vi "水温校准.vi"() -> ()   [LabVIEW 2016, in "斯坦道多参数.lvlib"]
uses:
  <vilib>/Utility/config.llb/NI_LVConfig.lvlib
panel:
  in  "补偿后温度值":dbl
  out "电极温度读值":dbl
  in  "温度偏移补偿":dbl
  in  "温度电极选择":enum16{"pH电极", "电导率电极", "溶解氧电极", "浊度电极"}(ring)
  # "温度电极设定"
  # "℃"
  # "℃"
  # "℃"
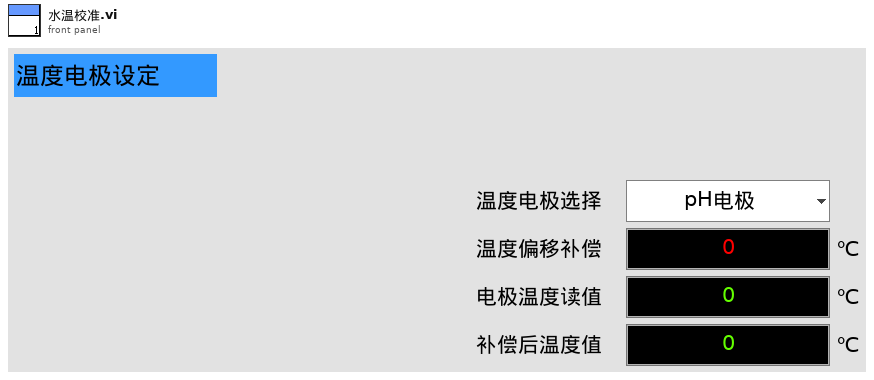
[diagram p1: front panel]
types:
  T1 = typedef "NI_LVConfig.lvlib/Config Data RefNum.ctl" = refnum<k1>
  T2 = cluster{"pH探头选择":u16, "DO探头选择":u16, "电导率探头选择":u16, "浊度探头选择":u16, "叶绿素a探头选择":u16, "蓝绿藻探头选择":u16, "orp探头选择":u16}
  T3 = cluster{"报警码":u16, "pH数值":sgl, "0X0003_NC":sgl, "温度数据":sgl, "pH原始信号 mv":sgl, "0X0009_NC":string, "产品名称":string, "序列号":string, "硬件版本":string, "软件版本":string, "通讯地址":u16, "波特率":u16, "设备类型":u16, "0X0026_NC":string, "第一点原始数据":sgl, "第一点校准数据":sgl, "第二点原始数据":sgl, "第二点校准数据":sgl, "探头校准命令":u16, "温度校准参数":sgl, "温度校准命令":u16}
  T4 = cluster{"报警码":u16, "电导率数据（uS/cm）":sgl, "0x0003 NC":sgl, "温度数据":sgl, "电导率原始信号电阻":sgl, "当前量程":u16, "温度补偿系数":sgl, "0X0009_NC":string, "产品名称":string, "序列号":string, "硬件版本":string, "软件版本":string, "通讯地址":u16, "波特率":u16, "设备类型":u16, "0X0026_NC":string, "第一点原始数据":sgl, "第一点校准数据":sgl, "0X0035_NC":sgl, "0X0037_NC":sgl, "探头校准命令":u16, "温度校准参数":sgl, "温度校准命令":u16}
  T5 = cluster{"报警码":u16, "溶解氧数值（mg/L）":sgl, "溶解氧数据（%）":sgl, "温度数据":sgl, "溶解氧原始信号 nA":sgl, "大气压力":sgl, "盐度":sgl, "0X0009_NC":string, "产品名称":string, "序列号":string, "硬件版本":string, "软件版本":string, "通讯地址":u16, "波特率":u16, "设备类型":u16, "0X0026_NC":string, "第一点原始数据":sgl, "第一点校准数据":sgl, "第二点原始数据":sgl, "第二点校准数据":sgl, "探头校准命令":u16, "温度校准参数":sgl, "温度校准命令":u16}
  T6 = cluster{"报警码":u16, "浊度数值 NTU":sgl, "温度数据":sgl, "原始光强数值":u16, "量程":u16, "平均次数":u16, "清扫模式":u16, "清扫次数":u16, "清扫间隔分钟":u16, "0X000B_NC":string, "产品名称":string, "序列号":string, "硬件版本":string, "软件版本":string, "通讯地址":u16, "波特率":u16, "设备类型":u16, "0X0026_NC":string, "校准量程":u16, "第一点原始光强":u16, "第一点校准数据":sgl, "第二点原始光强":u16, "第二点校准数据":sgl, "第三点原始光强":u16, "第三点校准数据":sgl, "探头校准命令":u16, "温度校准参数":sgl, "温度校准命令":u16}
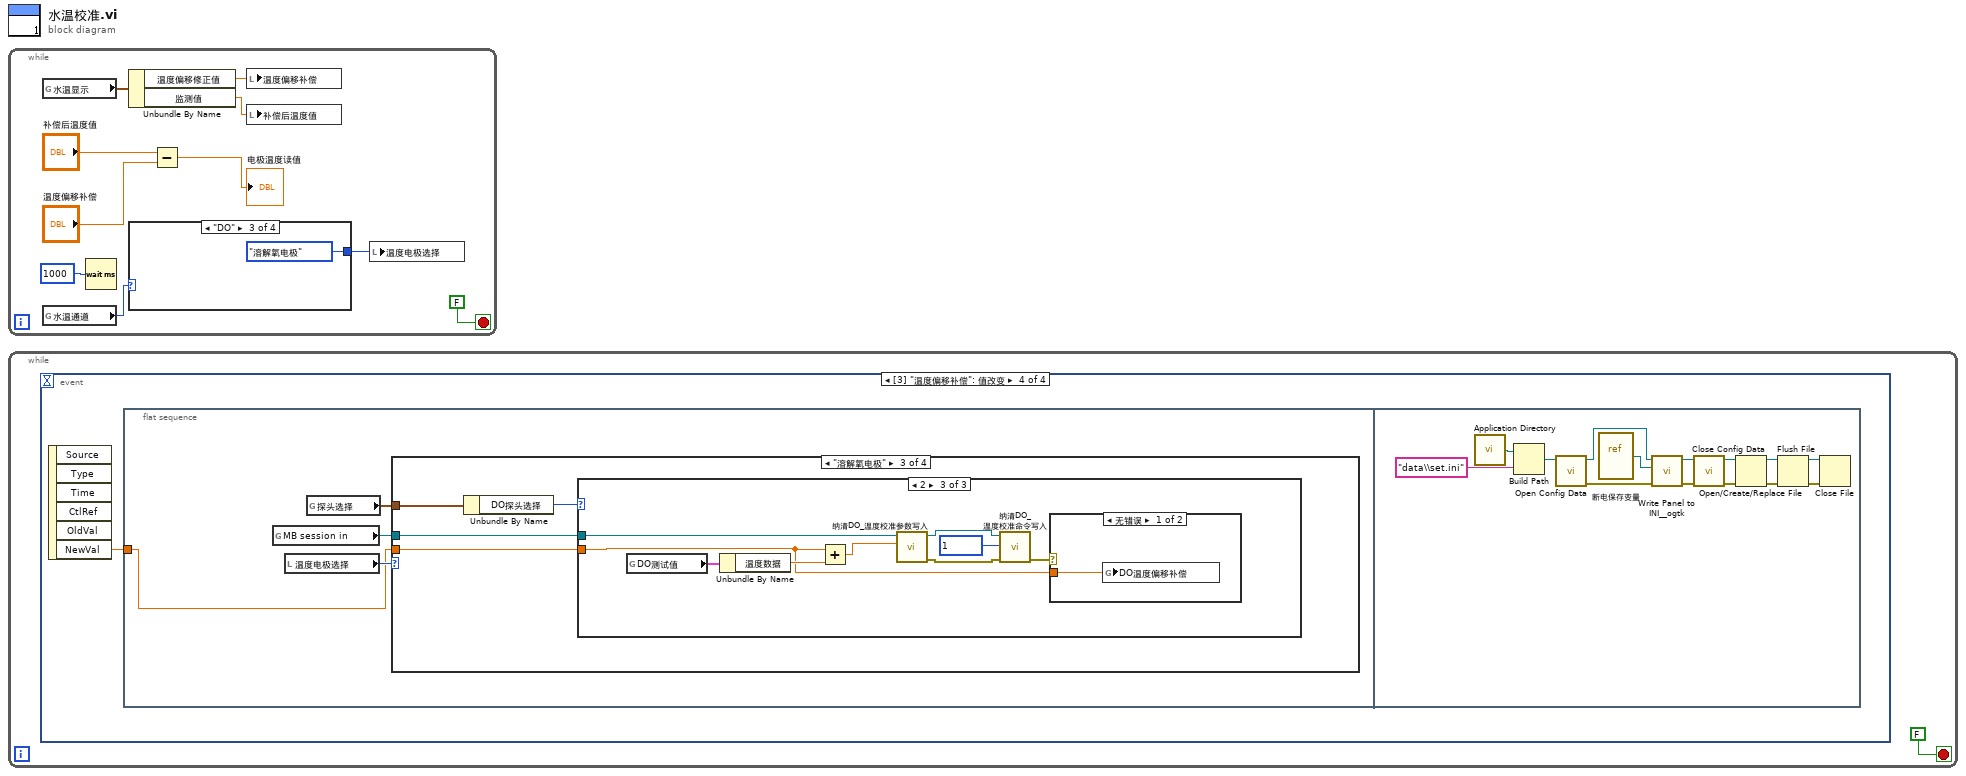
[diagram p0: block diagram]
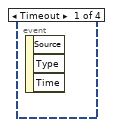
[diagram p2: hidden frame]
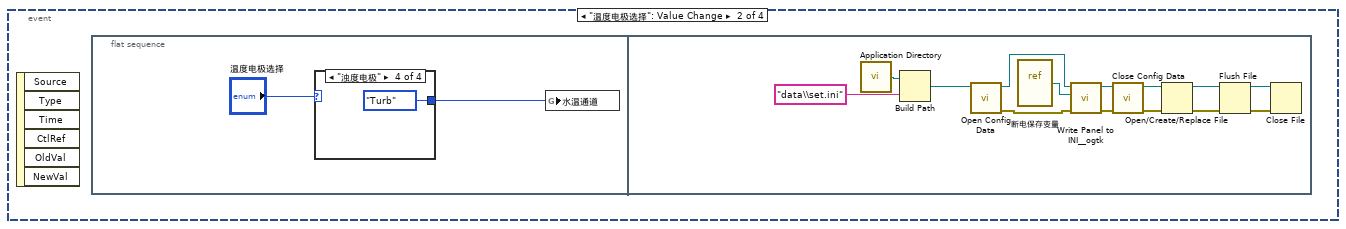
[diagram p3: hidden frame]
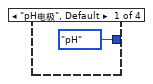
[diagram p4: hidden frame]
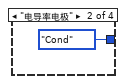
[diagram p5: hidden frame]
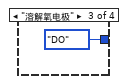
[diagram p6: hidden frame]
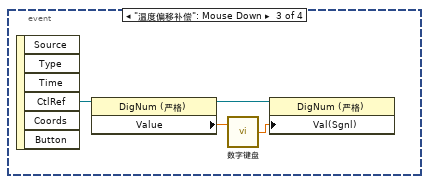
[diagram p7: hidden frame]
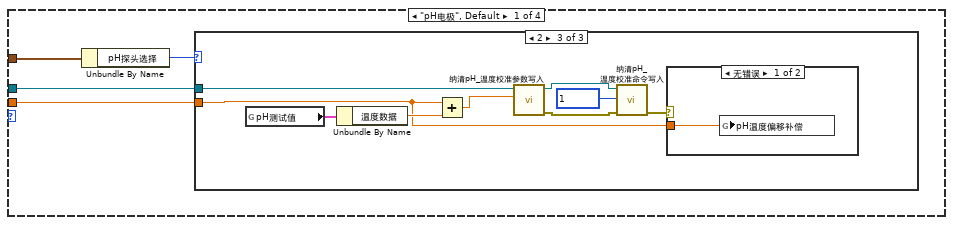
[diagram p8: hidden frame]
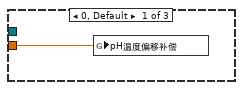
[diagram p9: hidden frame]
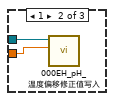
[diagram p10: hidden frame]
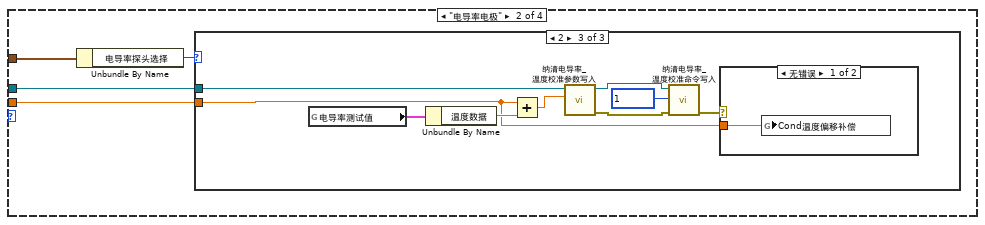
[diagram p12: hidden frame]
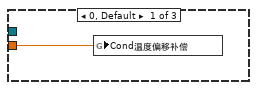
[diagram p13: hidden frame]
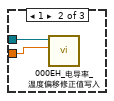
[diagram p14: hidden frame]
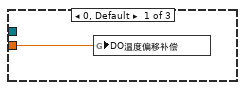
[diagram p16: hidden frame]
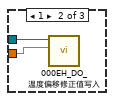
[diagram p17: hidden frame]
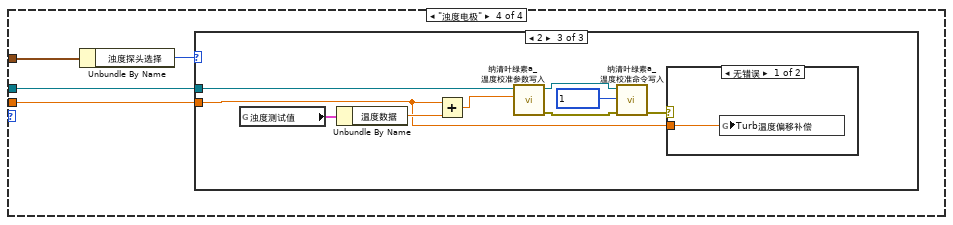
[diagram p19: hidden frame]
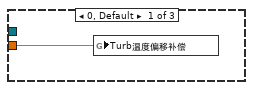
[diagram p20: hidden frame]
diagram:
  n1 = while {
    stop <- FALSE stop-if-true
    n2 = global read "多参数全局变量.vi" "水温显示"() -> (w1:cluster{"CH":u16, "监测值":dbl, "温度偏移修正值":sgl})
    n3 = global read "断电保存变量.vi" "水温通道"() -> (w3:enum16{"pH", "Cond", "DO", "Turb"})
    n4 = Wait (ms)(milliseconds to wait=u32 1000 ("等待时间（毫秒）")) -> ()  [unwired: 1 out]
    n5 = Unbundle By Name(w1) -> ("温度偏移修正值"=w5:sgl, "监测值"=w4:dbl)
    n6 = case shown="\"DO\"" w3 {
      tunnel: [enum16{"pH电极", "电导率电极", "溶解氧电极", "浊度电极"}."pH电极" ("温度电极选择") enum16{"pH电极", "电导率电极", "溶解氧电极", "浊度电极"}."电导率电极" ("温度电极选择") enum16{"pH电极", "电导率电极", "溶解氧电极", "浊度电极"}."溶解氧电极" ("温度电极选择") enum16{"pH电极", "电导率电极", "溶解氧电极", "浊度电极"}."浊度电极" ("温度电极选择")] -> w2
      frame "pH", Default {
      }
      frame "Cond" {
      }
      frame "DO" {
      }
      frame "Turb" {
      }
    }
    n7 = Subtract(x="补偿后温度值", y="温度偏移补偿") -> (x-y=→"电极温度读值":dbl)
    n8 = local write "温度偏移补偿"(w5) -> ()
    n9 = local write "补偿后温度值"(w4) -> ()
    n10 = local write "温度电极选择"(w2) -> ()
  }
  n11 = while {
    stop <- FALSE stop-if-true
    n12 = event shown="[3] \"温度偏移补偿\": 值改变" {
      selector: _ -> [_ _ _ _]
      dyn-events: _ -> [_ _ _ _]
      timeout: _ -> [_ _ _ _]
      event Timeout {
        n13 = event-data() -> ()  [unwired: 1 in, 3 out]
      }
      event "温度电极选择": Value Change {
        n14 = event-data() -> ()  [unwired: 1 in, 6 out]
        n15 = flat-sequence {
          frame #0 {
            n16 = case shown="\"浊度电极\"" "温度电极选择" {
              tunnel: [enum16{"pH", "Cond", "DO", "Turb"}."pH" ("水温通道") enum16{"pH", "Cond", "DO", "Turb"}."Cond" ("水温通道") enum16{"pH", "Cond", "DO", "Turb"}."DO" ("水温通道") enum16{"pH", "Cond", "DO", "Turb"}."Turb" ("水温通道")] -> w17
              frame "pH电极", Default {
              }
              frame "电导率电极" {
              }
              frame "溶解氧电极" {
              }
              frame "浊度电极" {
              }
            }
            n17 = global write "断电保存变量.vi" "水温通道"(w17) -> ()
          }
          frame #1 {
            n18 = call <vilib>:"Application Directory.vi"() -> ("Application Directory"=w31:path)
            n19 = Build Path(base path=w31, name or relative path="data\\set.ini" ("名称或相对路径")) -> (appended path=w30:path)
            n20 = call <vilib>:"Open Config Data.vi"("configuration file path"=w30) -> ("error out"=w34:errorcluster, "refnum"=w35:T1)  [unwired: 8 in, 1 out]
            n21 = vi-ref "断电保存变量.vi"() -> (w28:refnum<vi>)
            n22 = call <userlib>:"Write Panel to INI__ogtk.vi"("error in (no error)"=w34, "VI ref"=w28, "refnum"=w35) -> ("error out"=w32:errorcluster, "refnum out"=w33:T1)  [unwired: 7 in]
            n23 = call <vilib>:"Close Config Data.vi"("error in (no error)"=w32, "refnum"=w33) -> ("error out"=w24:errorcluster, "file path"=w25:path)  [unwired: 8 in]
            n24 = Open/Create/Replace File(file path (use dialog)=w25, error in=w24) -> (refnum out=w26:refnum<file>, error out=w27:errorcluster)  [unwired: 4 in, 1 out]
            n25 = Flush File(refnum=w26, error in=w27) -> (refnum out=w22:refnum<file>, error out=w23:errorcluster)
            n26 = Close File(refnum=w22, error in=w23) -> ()  [unwired: 2 out]
          }
        }
      }
      event "温度偏移补偿": Mouse Down {
        n27 = event-data() -> ("CtlRef"=w39:refnum<vi>)  [unwired: 1 in, 5 out]
        n28 = property class="DigNum (严格)"(reference=w39) -> (reference out=w36:refnum<vi>, "Value"=w38:dbl)  [unwired: 1 in, 1 out]
        n29 = call "数字键盘.vi"("OldNumber"=w38) -> ("NewNumber"=w37:dbl)  [unwired: 1 in]
        n30 = property class="DigNum (严格)"(reference=w36, "Val(Sgnl)"=w37) -> ()  [unwired: 1 in, 2 out]
      }
      event "温度偏移补偿": Value Change {
        n31 = event-data() -> ("NewVal"=w40:dbl)  [unwired: 1 in, 5 out]
        n32 = flat-sequence {
          tunnel: w40 -> [w43]
          frame #0 {
            n33 = global read "多参数全局变量.vi" "MB session in"() -> (w42:refnum<class "MB_Master.lvclass">)
            n34 = local read "温度电极选择"() -> (w44:enum16{"pH电极", "电导率电极", "溶解氧电极", "浊度电极"})
            n35 = global read "断电保存变量.vi" "探头选择"() -> (w41:T2)
            n36 = case shown="\"溶解氧电极\"" w44 {
              tunnel: w43 -> [w48 w65 w82 w99]
              tunnel: w42 -> [w47 w64 w79 w96]
              tunnel: w41 -> [w46 w63 w81 w98]
              frame "pH电极", Default {
                n37 = Unbundle By Name(w46) -> ("pH探头选择"=w45:u16)
                n38 = case shown="2" w45 {
                  tunnel: w48 -> [w49 w51 w52]
                  tunnel: w47 -> [_ w50 w54]
                  frame 0, Default {
                    n39 = global write "断电保存变量.vi" "pH温度偏移补偿"(w49) -> ()
                  }
                  frame 1 {
                    n40 = call "000EH_pH_温度偏移修正值写入.vi"("数值"=w51, "MB session in"=w50) -> ()  [unwired: 8 in, 2 out]
                  }
                  frame 2 {
                    n41 = global read "纳清过程全局变量.vi" "pH测试值"() -> (w60:T3)
                    n42 = Unbundle By Name(w60) -> ("温度数据"=w59:sgl)
                    n43 = Add(x=w52, y=w59) -> (x+y=w55:dbl)
                    n44 = call "纳清pH_温度校准参数写入.vi"("数值"=w55, "MB session in"=w54) -> ("error out"=w56:errorcluster, "MB session out"=w57:refnum<class "MB_Master.lvclass">)  [unwired: 8 in]
                    n45 = call "纳清pH_温度校准命令写入.vi"("error in (no error)"=w56, "数值"=u16 1 ("starting address"), "MB session in"=w57) -> ("error out"=w53:errorcluster)  [unwired: 7 in, 1 out]
                    n46 = case shown="无错误" w53 {
                      tunnel: w52 -> [w61 _]
                      frame No Error {
                        n47 = global write "断电保存变量.vi" "pH温度偏移补偿"(w61) -> ()
                      }
                      frame Error {
                      }
                    }
                  }
                }
              }
              frame "电导率电极" {
                n48 = Unbundle By Name(w63) -> ("电导率探头选择"=w62:u16)
                n49 = case shown="2" w62 {
                  tunnel: w65 -> [w66 w68 w69]
                  tunnel: w64 -> [_ w67 w74]
                  frame 0, Default {
                    n50 = global write "断电保存变量.vi" "Cond温度偏移补偿"(w66) -> ()
                  }
                  frame 1 {
                    n51 = call "000EH_电导率_温度偏移修正值写入.vi"("数值"=w68, "MB session in"=w67) -> ()  [unwired: 8 in, 2 out]
                  }
                  frame 2 {
                    n52 = global read "纳清过程全局变量.vi" "电导率测试值"() -> (w73:T4)
                    n53 = Unbundle By Name(w73) -> ("温度数据"=w72:sgl)
                    n54 = Add(x=w69, y=w72) -> (x+y=w71:dbl)
                    n55 = call "纳清电导率_温度校准参数写入.vi"("数值"=w71, "MB session in"=w74) -> ("error out"=w77:errorcluster, "MB session out"=w76:refnum<class "MB_Master.lvclass">)  [unwired: 8 in]
                    n56 = call "纳清电导率_温度校准命令写入.vi"("error in (no error)"=w77, "数值"=u16 1 ("starting address"), "MB session in"=w76) -> ("error out"=w70:errorcluster)  [unwired: 7 in, 1 out]
                    n57 = case shown="无错误" w70 {
                      tunnel: w69 -> [w78 _]
                      frame No Error {
                        n58 = global write "断电保存变量.vi" "Cond温度偏移补偿"(w78) -> ()
                      }
                      frame Error {
                      }
                    }
                  }
                }
              }
              frame "溶解氧电极" {
                n59 = Unbundle By Name(w81) -> ("DO探头选择"=w80:u16)
                n60 = case shown="2" w80 {
                  tunnel: w82 -> [w83 w84 w86]
                  tunnel: w79 -> [_ w85 w91]
                  frame 0, Default {
                    n61 = global write "断电保存变量.vi" "DO温度偏移补偿"(w83) -> ()
                  }
                  frame 1 {
                    n62 = call "000EH_DO_温度偏移修正值写入.vi"("数值"=w84, "MB session in"=w85) -> ()  [unwired: 8 in, 2 out]
                  }
                  frame 2 {
                    n63 = global read "纳清过程全局变量.vi" "DO测试值"() -> (w90:T5)
                    n64 = Unbundle By Name(w90) -> ("温度数据"=w89:sgl)
                    n65 = Add(x=w86, y=w89) -> (x+y=w88:dbl)
                    n66 = call "纳清DO_温度校准参数写入.vi"("数值"=w88, "MB session in"=w91) -> ("error out"=w94:errorcluster, "MB session out"=w93:refnum<class "MB_Master.lvclass">)  [unwired: 8 in]
                    n67 = call "纳清DO_温度校准命令写入.vi"("error in (no error)"=w94, "数值"=u16 1 ("starting address"), "MB session in"=w93) -> ("error out"=w87:errorcluster)  [unwired: 7 in, 1 out]
                    n68 = case shown="无错误" w87 {
                      tunnel: w86 -> [w95 _]
                      frame No Error {
                        n69 = global write "断电保存变量.vi" "DO温度偏移补偿"(w95) -> ()
                      }
                      frame Error {
                      }
                    }
                  }
                }
              }
              frame "浊度电极" {
                n70 = Unbundle By Name(w98) -> ("浊度探头选择"=w97:u16)
                n71 = case shown="2" w97 {
                  tunnel: w99 -> [w100 w102 w103]
                  tunnel: w96 -> [_ w101 w107]
                  frame 0, Default {
                    n72 = global write "断电保存变量.vi" "Turb温度偏移补偿"(w100) -> ()
                  }
                  frame 1 {
                    n73 = call "000EH_浊度_温度偏移修正值写入.vi"("数值"=w102, "MB session in"=w101) -> ()  [unwired: 8 in, 2 out]
                  }
                  frame 2 {
                    n74 = global read "纳清过程全局变量.vi" "浊度测试值"() -> (w111:T6)
                    n75 = Unbundle By Name(w111) -> ("温度数据"=w106:sgl)
                    n76 = Add(x=w103, y=w106) -> (x+y=w105:dbl)
                    n77 = call "纳清叶绿素a_温度校准参数写入.vi"("数值"=w105, "MB session in"=w107) -> ("error out"=w108:errorcluster, "MB session out"=w109:refnum<class "MB_Master.lvclass">)  [unwired: 8 in]
                    n78 = call "纳清叶绿素a_温度校准命令写入.vi"("error in (no error)"=w108, "数值"=u16 1 ("starting address"), "MB session in"=w109) -> ("error out"=w104:errorcluster)  [unwired: 7 in, 1 out]
                    n79 = case shown="无错误" w104 {
                      tunnel: w103 -> [w112 _]
                      frame No Error {
                        n80 = global write "断电保存变量.vi" "Turb温度偏移补偿"(w112) -> ()
                      }
                      frame Error {
                      }
                    }
                  }
                }
              }
            }
          }
          frame #1 {
            n81 = call <vilib>:"Application Directory.vi"() -> ("Application Directory"=w122:path)
            n82 = Build Path(base path=w122, name or relative path="data\\set.ini" ("名称或相对路径")) -> (appended path=w121:path)
            n83 = call <vilib>:"Open Config Data.vi"("configuration file path"=w121) -> ("error out"=w125:errorcluster, "refnum"=w126:T1)  [unwired: 8 in, 1 out]
            n84 = vi-ref "断电保存变量.vi"() -> (w119:refnum<vi>)
            n85 = call <userlib>:"Write Panel to INI__ogtk.vi"("error in (no error)"=w125, "VI ref"=w119, "refnum"=w126) -> ("error out"=w123:errorcluster, "refnum out"=w124:T1)  [unwired: 7 in]
            n86 = call <vilib>:"Close Config Data.vi"("error in (no error)"=w123, "refnum"=w124) -> ("error out"=w115:errorcluster, "file path"=w116:path)  [unwired: 8 in]
            n87 = Open/Create/Replace File(file path (use dialog)=w116, error in=w115) -> (refnum out=w117:refnum<file>, error out=w118:errorcluster)  [unwired: 4 in, 1 out]
            n88 = Flush File(refnum=w117, error in=w118) -> (refnum out=w113:refnum<file>, error out=w114:errorcluster)
            n89 = Close File(refnum=w113, error in=w114) -> ()  [unwired: 2 out]
          }
        }
      }
    }
  }
